vi "Error Query.vi"(7 "Channel (0: SIM900)":i32(ring) items=["SIM900", "1", "2", "3", "4", "5", "6", "7", "8", "9", "A", "B", "C", "D"], 8 "error in (no error)":errorcluster, 11 "VISA resource name":refnum<visa-resource-name>) -> (0 "error out":errorcluster, 1 "Error Message":string, 2 "Error Code":i32, 3 "VISA resource name out":refnum<visa-resource-name>)   [LabVIEW 2019, in "Stanford Research SIM900 Series.lvlib"]
doc: "Queries the instrument for any errors in the instrument's error queue. It will continue to read errors until all errors have been read from the instrument. Any errors will be returned in the <B>error out</B> control.\n\n<B>Note:</B>\nThis VI is called automatically by most driver VIs so it is not usually necessary to call this in an application."
uses:
  Stanford Research SIM900 Series.lvlib
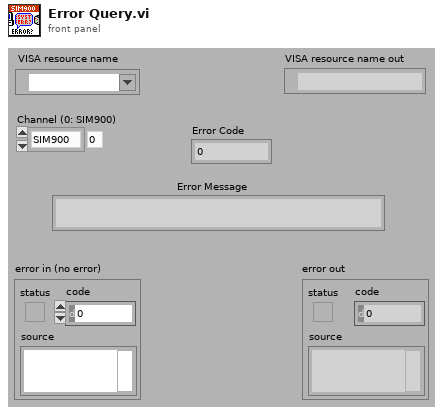
[diagram p1: front panel]
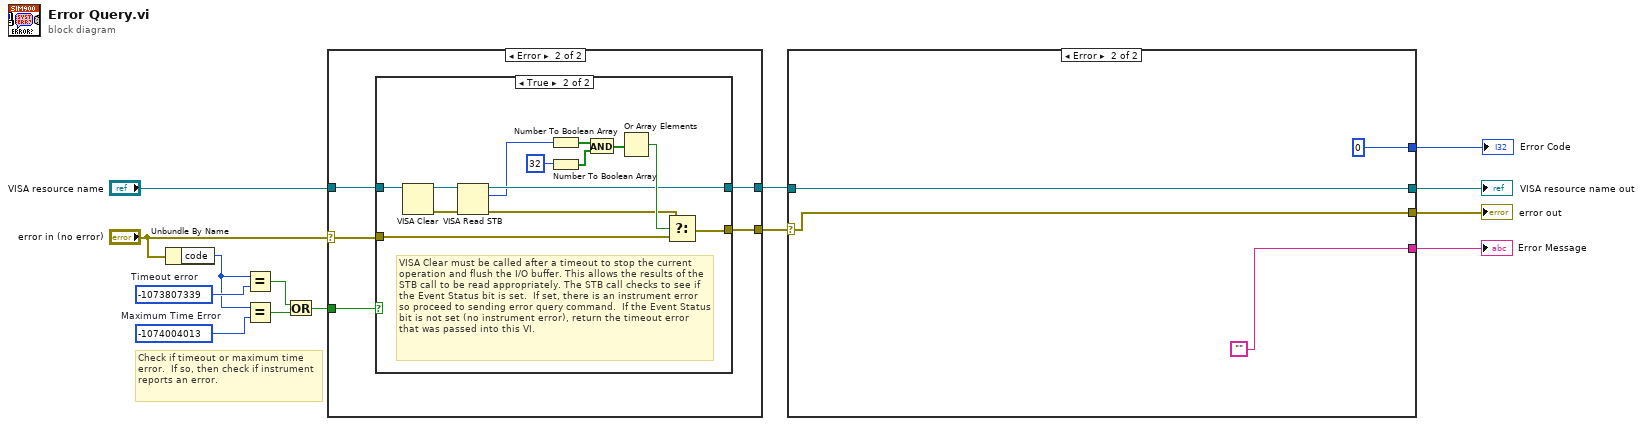
[diagram p0: block diagram]
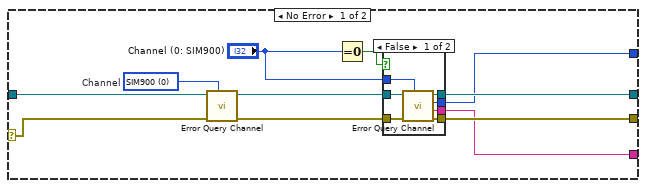
[diagram p4: hidden frame]
diagram:
  w6 = -1074004013  # Maximum Time Error
  w8 = -1073807339  # Timeout error
  # "Check if timeout or maximum time error.  If so, then check if instrument reports an error."
  n1 = Unbundle By Name("error in (no error)") -> ("code"=w7:i32)
  n2 = Equal?(x=w7, y=w8) -> (x = y?=w4:bool)
  n3 = Equal?(x=w7, y=w6) -> (x = y?=w5:bool)
  n4 = Or(x=w4, y=w5) -> (x .or. y?=w3:bool)
  n5 = case shown="Error" "error in (no error)" {
    selector: "error in (no error)" -> [w15 w19]
    tunnel: "VISA resource name" -> [w16 w21]
    tunnel: [w16 w20] -> w10
    tunnel: [w15 w18] -> w11
    tunnel: w3 -> [_ w17]
    frame No Error {
    }
    frame Error {
      n6 = case shown="True" w17 {
        tunnel: w21 -> [w23 w29]
        tunnel: [w23 w26] -> w20
        tunnel: w19 -> [w22 w32]
        tunnel: [w22 w31] -> w18
        frame False {
          # "Error code not a timeout, so best to pass on to user."
        }
        frame True {
          # "VISA Clear must be called after a timeout to stop the current operation and flush the I/O buffer. This allows the results of the  STB call to be read appropriately. The STB call checks to see if the Event Status bit is set.  If set, there is an instrument error so proceed to sending error query command.  If the Event Status bit is not set (no instrument error), return the timeout error that was passed into this VI."
          n7 = VISA Clear(VISA resource name=w29) -> (VISA resource name out=w28:refnum<visa-resource-name>, error out=w27:errorcluster)  [unwired: 1 in]
          n8 = VISA Read STB(8:w27, 11:w28) -> (0:w25:errorcluster, 2:w24:u16, 3:w26:refnum<visa-resource-name>)
          n9 = Number To Boolean Array(number=w24) -> (Boolean array=w33:bool[])
          n10 = Number To Boolean Array(number=32) -> (Boolean array=w35:bool[])
          n11 = And(x=w33, y=w35) -> (x .and. y?=w34:bool[])
          n12 = Or Array Elements(Boolean array=w34) -> (logical OR=w30:bool)
          n13 = Select(t=w25, s=w30, f=w32) -> (s? t:f=w31:errorcluster)
        }
      }
    }
  }
  n14 = case shown="Error" w11 {
    selector: w11 -> [w45 w58]
    tunnel: [w42 w60] -> w14
    tunnel: w10 -> [w47 w60]
    tunnel: [w43 w58] -> w13
    tunnel: [w40 ""] -> w12
    tunnel: [w41 0] -> w1
    frame No Error {
      w37 = 0 items=["SIM900", "1", "2", "3", "4", "5", "6", "7", "8", "9", "A", "B", "C", "D"]  # Channel
      n15 = call "Error Query Channel.vi"("Channel (0: SIM900)"=w37, "error in (no error)"=w45, "VISA resource name"=w47) -> ("error out"=w44:errorcluster, "VISA resource name out"=w46:refnum<visa-resource-name>)  [unwired: 5 in, 2 out]
      n16 = Equal To 0?(x="Channel (0: SIM900)") -> (x = 0?=w39:bool)
      n17 = case shown="False" w39 {
        tunnel: w46 -> [w54 w56]
        tunnel: w44 -> [w53 w55]
        tunnel: [w52 w55] -> w43
        tunnel: [w51 w56] -> w42
        tunnel: [w50 _] -> w41
        tunnel: [w49 _] -> w40
        tunnel: "Channel (0: SIM900)" -> [w48 _]
        frame False {
          n18 = call "Error Query Channel.vi"("Channel (0: SIM900)"=w48, "error in (no error)"=w53, "VISA resource name"=w54) -> ("error out"=w52:errorcluster, "Error Message"=w49:string, "Error Code"=w50:i32, "VISA resource name out"=w51:refnum<visa-resource-name>)  [unwired: 5 in]
        }
        frame True {
        }
      }
    }
    frame Error {
    }
  }
  "VISA resource name out" <- w14
  "error out" <- w13
  "Error Message" <- w12
  "Error Code" <- w1
